vi "bin xy graphv02.vi"(3 "Error Bar Type":T1(ring), 4 "interval":dbl=0.5, 5 "FIXED X INTERVAL?":bool=TRUE, 6 "Input Graph":cluster{"y vector":dbl[], "avg optspec":dbl[]}(graph) caption="Energy transmission energy meter") -> (0 "Array avgs and errors":dbl[][](array[numeric]), 1 "standard dev":dbl[](array[numeric]), 2 "Binned graph":cluster{"y vector":dbl[], "avg optspec":dbl[]}[](graph) caption="Energy transmission energy meter")   [LabVIEW 2009]
uses:
  <vilib>/gmath/statdist.llb/st_Percentiles (scalar).vi
  <vilib>/Analysis/NI_AALBase.lvlib
  <vilib>/gmath/NI_Gmath.lvlib
panel:
  out "mean":dbl format="%0.2f"
  out "y error high":dbl[](array[numeric])
  out "y error low":dbl[](array[numeric])
  out "Array":bool[](array[boolean])
  out "x/y":i32
  out "YZ 2":cluster{"y vector":dbl[], "avg optspec":dbl[]}[](graph) caption="Energy transmission energy meter"
  out "avgd y":dbl[](array[numeric])
  out "avgd x":dbl[](array[numeric])
  out "buckets":dbl[](array[numeric])
  out "min value":dbl
  out "max value":dbl
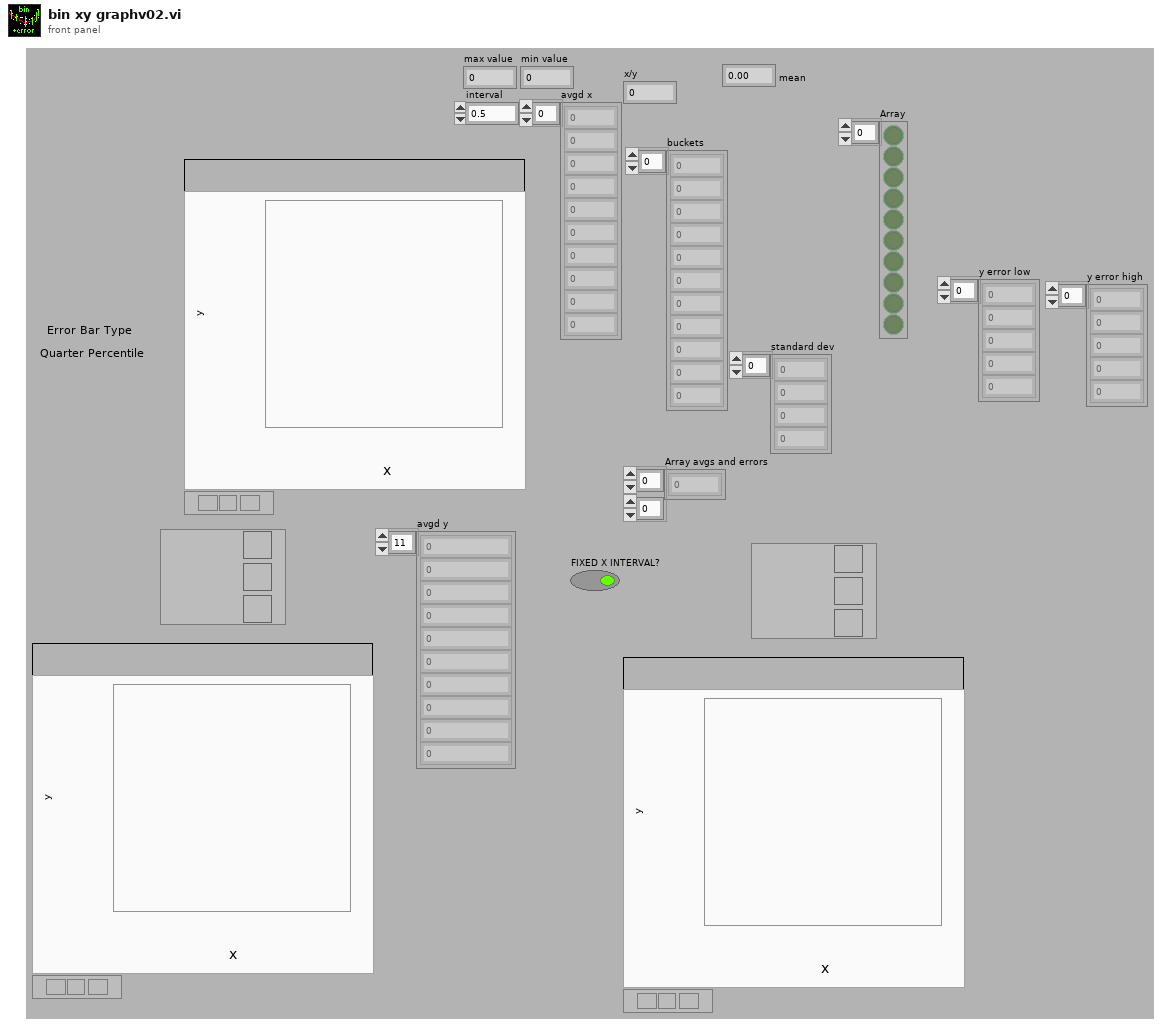
[diagram p1: front panel]
types:
  T1 = enum16{"Quarter Percentile", "Standard Deviation"}
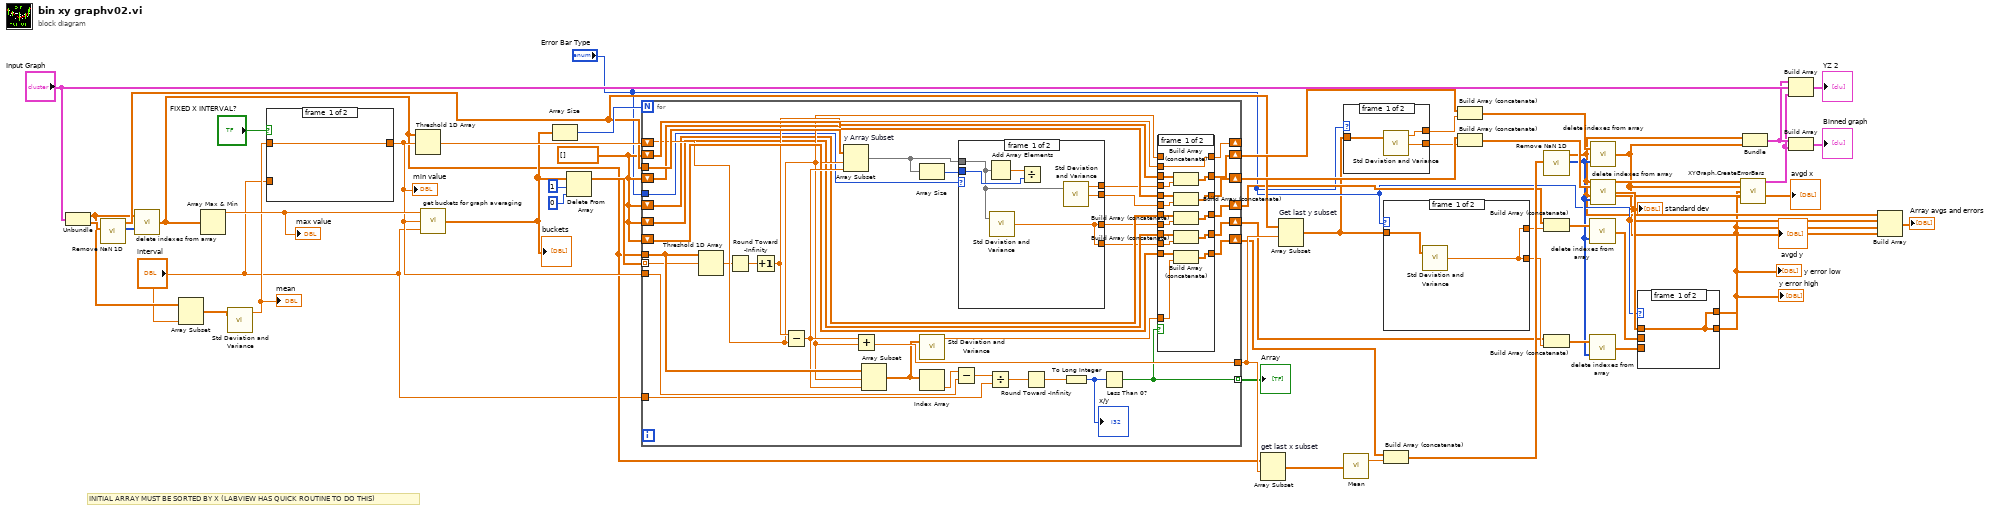
[diagram p0: block diagram]
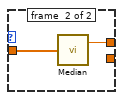
[diagram p2: hidden frame]
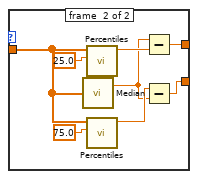
[diagram p3: hidden frame]
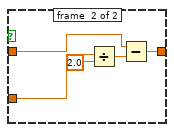
[diagram p5: hidden frame]
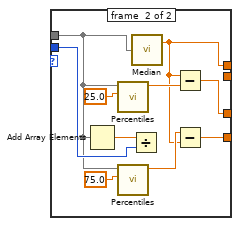
[diagram p6: hidden frame]
diagram:
  w14 = dbl[] [] ("avgd x")
  # "INITIAL ARRAY MUST BE SORTED BY X (LABVIEW HAS QUICK ROUTINE TO DO THIS)"
  n1 = Unbundle("Input Graph") -> ("y vector"=w4:dbl[], "avg optspec"=w28:dbl[])
  n2 = call "Remove NaN 1D.vi"("Array in"=w28) -> ("indexes removed"=w27:i32[], "Array out"=w24:dbl[])  [unwired: 9 out]
  n3 = call "delete indexes from array.vi"("indexes removed"=w27, "array in"=w4) -> ("array out"=w26:dbl[])
  n4 = Array Subset(array=w4, length="interval") -> (w3:dbl[])  [unwired: 1 in]
  n5 = Array Max & Min(array=w26) -> (max value=w52:dbl)  [unwired: 3 out]
  "max value" <- w52
  n6 = call <vilib>:"Std Deviation and Variance.vi"("X"=w3) -> ("mean"=w2:dbl)  [unwired: 1 in, 2 out]
  "mean" <- w2
  n7 = case shown="True" "FIXED X INTERVAL?" {
    tunnel: w2 -> [w53 w58]
    tunnel: [w53 w57] -> w35
    tunnel: "interval" -> [_ w56]
    frame #0 {
    }
    frame #1 {
      n8 = Divide(x=w56, y=2.0) -> (x/y=w54:dbl)
      n9 = Subtract(x=w58, y=w54) -> (x-y=w57:dbl)
    }
  }
  "min value" <- w35
  n10 = Threshold 1D Array(2:w35, 3:w26) -> (0:w50:dbl)  [unwired: 1 out]
  n11 = call "get buckets for graph averaging.vi"("interval"="interval", "Numeric"=w35, "Numeric 2"=w52) -> ("Array"=w46:dbl[])
  "buckets" <- w46
  n12 = Array Size(array=w46) -> (size(s)=w48:i32)
  n13 = Delete From Array(array=w46, length=1, index=0) -> (array with subset deleted=w47:dbl[])  [unwired: 1 out]
  n14 = for {
    N: w48 -> [_]
    tunnel: w26 -> [w95]
    tunnel: w24 -> [w92]
    shift-right: [w76] -> _
    shift-left: w50 -> [w74]
    tunnel: w47 -> [w94] mode=indexing
    tunnel: [w93] -> w43
    tunnel: "interval" -> [w90]
    tunnel: w35 -> [w86]
    tunnel: [w70] -> w37 mode=indexing
    shift-right: [w82] -> w33
    shift-left: w14 -> [w83]
    shift-right: [w80] -> w31
    shift-left: w14 -> [w79]
    shift-right: [w77] -> w36
    shift-left: w14 -> [w78]
    tunnel: "Error Bar Type" -> [w67]
    shift-right: [w66] -> w23
    shift-left: w14 -> [w64]
    shift-right: [w65] -> w20
    shift-left: w14 -> [w63]
    n15 = Threshold 1D Array(2:w94, 3:w95) -> (0:w73:dbl)  [unwired: 1 out]
    n16 = Round Toward -Infinity(1:w73) -> (0:w72:dbl)
    n17 = Increment(x=w72) -> (x+1=w75:dbl)
    n18 = Subtract(x=w75, y=w74) -> (x-y=w91:dbl)
    n19 = Array Subset "y Array Subset"(array=w92, index=w74, length=w91) -> (w68:dbl[])
    n20 = Add(x=w91, y=w74) -> (x+y=w93:dbl)
    n21 = Array Subset(array=w95, index=w74, length=w91) -> (w89:dbl[])
    n22 = Array Size(array=w68) -> (size(s)=w69:i32)
    n23 = call <vilib>:"Std Deviation and Variance.vi"("X"=w89) -> ("mean"=w81:dbl)  [unwired: 1 in, 2 out]
    n24 = Index Array(array=w89) -> (element=w87:dbl)  [unwired: 1 in]
    n25 = Subtract(x=w87, y=w86) -> (x-y=w85:dbl)
    n26 = case shown="\"Standard Deviation\", Default" w67 {
      tunnel: w68 -> [w98 w103]
      tunnel: [w101 w108] -> w62
      tunnel: [w101 w107] -> w61
      tunnel: w69 -> [w99 w110]
      tunnel: [w97 w102] -> w60
      tunnel: [w96 _] -> w59
      frame #0 {
        n27 = Add Array Elements(numeric array=w98) -> (sum=w100:dbl)
        n28 = call <vilib>:"Std Deviation and Variance.vi"("X"=w98) -> ("standard deviation"=w101:dbl)  [unwired: 1 in, 2 out]
        n29 = Divide(x=w100, y=w99) -> ()  [unwired: 1 out]
        n30 = call <vilib>:"Std Deviation and Variance.vi"("X"=w98) -> ("mean"=w97:dbl, "standard deviation"=w96:dbl)  [unwired: 1 in, 1 out]
      }
      frame #1 {
        n31 = Add Array Elements(numeric array=w103) -> (sum=w111:dbl)
        n32 = call-poly <vilib>:"Percentiles.vi"("p"=25.0, "x array"=w103) -> ("percentile"=w109:dbl)  [unwired: 9 out]
        n33 = call-poly <vilib>:"Percentiles.vi"("p"=75.0, "x array"=w103) -> ("percentile"=w106:dbl)  [unwired: 9 out]
        n34 = Divide(x=w111, y=w110) -> ()  [unwired: 1 out]
        n35 = call <vilib>:"Median.vi"("X"=w103) -> ("median"=w102:dbl)  [unwired: 1 out]
        n36 = Subtract(x=w102, y=w109) -> (x-y=w108:dbl)
        n37 = Subtract(x=w106, y=w102) -> (x-y=w107:dbl)
      }
    }
    n38 = Divide(x=w85, y=w90) -> (x/y=w88:dbl)
    n39 = Round Toward -Infinity(1:w88) -> (0:w84:dbl)
    n40 = To Long Integer(number=w84) -> (32bit integer=w71:i32)
    "x/y" <- w71
    n41 = Less Than 0?(x=w71) -> (x < 0?=w70:bool)
    n42 = case shown="False" w70 {
      tunnel: w83 -> [w127 w133]
      tunnel: [w125 w133] -> w82
      tunnel: w81 -> [w126 _]
      tunnel: [w122 w132] -> w80
      tunnel: w79 -> [w124 w132]
      tunnel: w60 -> [w123 _]
      tunnel: w78 -> [w118 w131]
      tunnel: [w121 w131] -> w77
      tunnel: w59 -> [w120 _]
      tunnel: [w119 w130] -> w76
      tunnel: w75 -> [w119 _]
      tunnel: w74 -> [_ w130]
      tunnel: [w117 w129] -> w66
      tunnel: [w116 w128] -> w65
      tunnel: w64 -> [w115 w129]
      tunnel: w63 -> [w114 w128]
      tunnel: w62 -> [w113 _]
      tunnel: w61 -> [w112 _]
      frame #0 {
        n43 = Build Array (concatenate)(w124, w123) -> (w122:dbl[])
        n44 = Build Array (concatenate)(w118, w120) -> (w121:dbl[])
        n45 = Build Array (concatenate)(w115, w113) -> (w117:dbl[])
        n46 = Build Array (concatenate)(w114, w112) -> (w116:dbl[])
        n47 = Build Array (concatenate)(w127, w126) -> (w125:dbl[])
      }
      frame #1 {
      }
    }
  }
  "Array" <- w37
  n48 = Array Subset "get last x subset"(array=w26, index=w43) -> (w42:dbl[])  [unwired: 1 in]
  n49 = Array Subset "Get last y subset"(array=w24, index=w43) -> (w12:dbl[])  [unwired: 1 in]
  n50 = case shown="\"Quarter Percentile\"" "Error Bar Type" {
    tunnel: w12 -> [w136 w138]
    tunnel: [w135 w137] -> w11
    tunnel: [w134 _] -> w10
    frame #0 {
      n51 = call <vilib>:"Std Deviation and Variance.vi"("X"=w136) -> ("mean"=w135:dbl, "standard deviation"=w134:dbl)  [unwired: 1 in, 1 out]
    }
    frame #1 {
      n52 = call <vilib>:"Median.vi"("X"=w138) -> ("median"=w137:dbl)  [unwired: 1 out]
    }
  }
  n53 = call <vilib>:"Mean.vi"("X"=w42) -> ("mean"=w41:dbl)  [unwired: 1 out]
  n54 = case shown="\"Quarter Percentile\"" "Error Bar Type" {
    tunnel: w12 -> [w140 w142]
    tunnel: [w139 w147] -> w22
    tunnel: [w139 w146] -> w21
    frame #0 {
      n55 = call <vilib>:"Std Deviation and Variance.vi"("X"=w140) -> ("standard deviation"=w139:dbl)  [unwired: 1 in, 2 out]
    }
    frame #1 {
      n56 = call <vilib>:"Median.vi"("X"=w142) -> ("median"=w141:dbl)  [unwired: 1 out]
      n57 = call-poly <vilib>:"Percentiles.vi"("p"=25.0, "x array"=w142) -> ("percentile"=w148:dbl)  [unwired: 9 out]
      n58 = call-poly <vilib>:"Percentiles.vi"("p"=75.0, "x array"=w142) -> ("percentile"=w145:dbl)  [unwired: 9 out]
      n59 = Subtract(x=w141, y=w148) -> (x-y=w147:dbl)
      n60 = Subtract(x=w145, y=w141) -> (x-y=w146:dbl)
    }
  }
  n61 = Build Array (concatenate)(w33, w41) -> (w32:dbl[])
  n62 = Build Array (concatenate)(w31, w11) -> (w30:dbl[])
  n63 = Build Array (concatenate)(w36, w10) -> (w29:dbl[])
  n64 = call "Remove NaN 1D.vi"("Array in"=w32) -> ("indexes removed"=w17:i32[], "Array out"=w9:dbl[])  [unwired: 9 out]
  "avgd x" <- w9
  n65 = Build Array (concatenate)(w23, w22) -> (w19:dbl[])
  n66 = Build Array (concatenate)(w20, w21) -> (w18:dbl[])
  n67 = call "delete indexes from array.vi"("indexes removed"=w17, "array in"=w19) -> ("array out"=w16:dbl[])
  n68 = call "delete indexes from array.vi"("indexes removed"=w17, "array in"=w18) -> ("array out"=w15:dbl[])
  n69 = call "delete indexes from array.vi"("indexes removed"=w17, "array in"=w30) -> ("array out"=w8:dbl[])
  "avgd y" <- w8
  n70 = call "delete indexes from array.vi"("indexes removed"=w17, "array in"=w29) -> ("array out"=w25:dbl[])
  "standard dev" <- w25
  n71 = case shown="\"Standard Deviation\", Default" "Error Bar Type" {
    tunnel: w25 -> [w149 _]
    tunnel: [w149 w150] -> w6
    tunnel: [w149 w151] -> w7
    tunnel: w16 -> [_ w151]
    tunnel: w15 -> [_ w150]
    frame #0 {
    }
    frame #1 {
    }
  }
  "y error low" <- w7
  "y error high" <- w6
  n72 = call "XYGraph.CreateErrorBars.vi"("X"=w9, "Y"=w8, "error low"=w7, "error high"=w6) -> ("error bar plot"=w39:cluster{dbl[], dbl[]})  [unwired: 11 out]
  n73 = Bundle("Array out"=w9, "array out"=w8) -> (w40:cluster{"Array out":dbl[], "array out":dbl[]})  [unwired: 1 out]
  n74 = Build Array(w40, "Input Graph", w39) -> (→"YZ 2":cluster{"y vector":dbl[], "avg optspec":dbl[]}[])
  n75 = Build Array(w40, w39) -> (→"Binned graph":cluster{"Array out":dbl[], "array out":dbl[]}[])
  n76 = Build Array(w9, w8, w7, w6) -> (→"Array avgs and errors":dbl[][])
